vi "Start Command.vi"(8 "error in (no error)":errorcluster, 9 "Command Name":string, 10 "Robot Actors.lvlib:Command.lvlib:Command.lvclass":refnum<class "Command.lvclass">, 11 "No Command in":refnum<class "No Command.lvclass">) -> (0 "error out":errorcluster, 3 "No Command out":refnum<class "No Command.lvclass">)   [LabVIEW 2013, in "Robot Actors.lvlib" / "Command Processor.lvlib" / "No Command.lvclass"]
uses:
  No Command.lvclass
  Command/Command Class/Command.lvclass
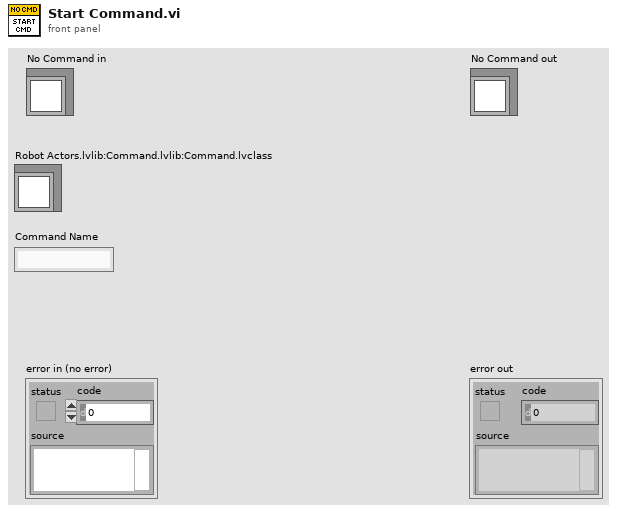
[diagram p1: front panel]
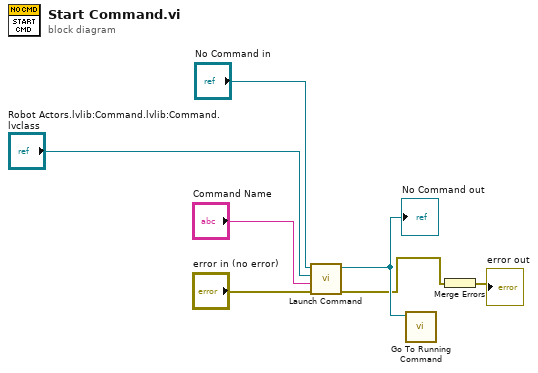
[diagram p0: block diagram]
diagram:
  n1 = call-dynamic "Launch Command.vi"("error in (no error)"="error in (no error)", "Command Name"="Command Name", "Robot Actors.lvlib:Command.lvlib:Command.lvclass"="Robot Actors.lvlib:Command.lvlib:Command.lvclass", "Command Processor in"="No Command in") -> ("error out"=w1:errorcluster, "Command Processor out"=w2:refnum<class "No Command.lvclass">)  [unwired: 6 in]
  "No Command out" <- w2
  n2 = call-dynamic "Go To Running Command.vi"("Command Processor in"=w2) -> ()  [unwired: 9 in, 2 out]
  n3 = Merge Errors(w1) -> (→"error out":errorcluster)
